vi "ZLIB Enumerate File Contents Old__ogtk.vi"(8 "error in (no error)":errorcluster, 11 "unzip Refnum":T2) -> (0 "error out":errorcluster, 1 "file infos":T1[](array[typedef]) {"file timestamp" format="%<%H:%M:%S\n%d/%m/%Y>T"; "external fa" format="%.0x"; "internal fa" format="%.0x"; "crc" format="%.0x"}, 2 "file names":string[](array[string]), 3 "unzip Refnum out":T2, 4 "file comments":string[](array[string]), 5 "extra data":string[](array[string]), 6 "global comment":string)   [LabVIEW 2020]
doc: "Lists all the information contained in the file of an unzip session."
uses:
  <userlib>/_OpenG.lib/lvzip/lvzip.llb/ZLIB Unzip Handle__ogtk.ctl
  <userlib>/_OpenG.lib/lvzip/lvzip.llb/ZLIB File Info Old__ogtk.ctl
panel:
  in  "file info":T1 {"file timestamp" format="%<%H:%M:%S\n%d/%m/%Y>T"; "external fa" format="%.0x"; "internal fa" format="%.0x"; "crc" format="%.0x"}
  # "Please visit http://www.OpenG.org to learn about the\nOpen Source LabVIEW software movement.\n\nNOTICE -- YOU MUST LEAVE THIS NOTICE IN PLACE.  PER THE TERMS OF THE LICENSE BELOW, YOU MAY SUBLICENSE THIS SOFTWARE \nIN ANY WAY THAT DOES NOT CONFLICT WITH THIS LICENSE.\n\n### BSD License (http://www.opensource.org/licenses/bsd-license.php) Begin ###\n \nCopyright (C) 2002-2004 Rolf Kalbermatter rolf.kalbermatter@citeng.com\nCopyright (C) 2002 Jim Kring jim@jimkring.com\n\nAll rights reserved.\n\nRedistribution and use in source and binary forms, with or without modification, are permitted provided that the following conditions are met:\n\n    * Redistributions of source code must retain the above copyright notice, this list of conditions and the following disclaimer.\n    * Redistributions in binary form must reproduce the above copyright notice, this list of conditions and the following disclaimer in the \n       documentation and/or other materials provided with the distribution.\n    * Neither the name of SciWare, James Kring, Inc., nor the names of its contributors may be used to endorse or promote products derived \n       from this software without specific prior written permission.\n\nTHIS SOFTWARE IS PROVIDED BY THE COPYRIGHT HOLDERS AND CONTRIBUTORS \"AS IS\" AND ANY EXPRESS OR IMPLIED WARRANTIES, \nINCLUDING, BUT NOT LIMITED TO, THE IMPLIED WARRANTIES OF MERCHANTABILITY AND FITNESS FOR A PARTICULAR PURPOSE ARE \nDISCLAIMED. IN NO EVENT SHALL THE COPYRIGHT OWNER OR CONTRIBUTORS BE LIABLE FOR ANY DIRECT, INDIRECT, INCIDENTAL,\n SPECIAL, EXEMPLARY, OR CONSEQUENTIAL DAMAGES (INCLUDING, BUT NOT LIMITED TO, PROCUREMENT OF SUBSTITUTE GOODS OR \nSERVICES; LOSS OF USE, DATA, OR PROFITS; OR BUSINESS INTERRUPTION) HOWEVER CAUSED AND ON ANY THEORY OF LIABILITY, \nWHETHER IN CONTRACT, STRICT LIABILITY, OR TORT (INCLUDING NEGLIGENCE OR OTHERWISE) ARISING IN ANY WAY OUT OF THE USE \nOF THIS SOFTWARE, EVEN IF ADVISED OF THE POSSIBILITY OF SUCH DAMAGE.\n\n### BSD License End ###"
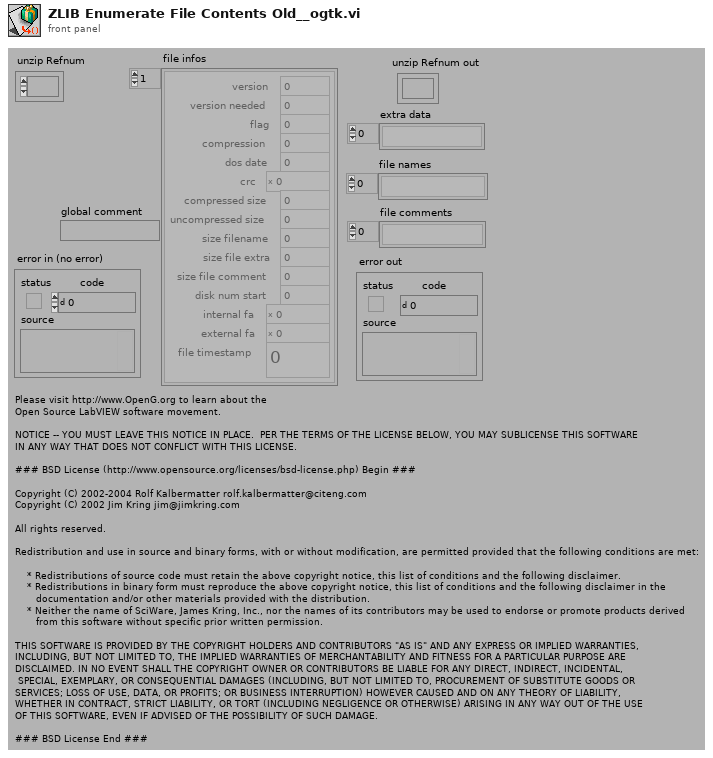
[diagram p1: front panel]
types:
  T1 = typedef "ZLIB File Info Old__ogtk.ctl" = cluster{"version":u32, "version needed":u32, "flag":u32, "compression":u32, "dos date":u32, "crc":u32, "compressed size":u32, "uncompressed size":u32, "size filename":u32, "size file extra":u32, "size file comment":u32, "disk num start":u32, "internal fa":u32, "external fa":u32, "file timestamp":u32}
  T2 = typedef "ZLIB Unzip Handle__ogtk.ctl" = refnum<k1>
  T3 = typedef "ZLIB File Info__ogtk.ctl" = cluster{"version":u32, "version needed":u32, "encrypted":bool, "flag":u32, "compression":i32, "dos date":u32, "crc":u32, "compressed size":u32, "uncompressed size":u32, "extra info":string, "file comment":string, "disk num start":u32, "internal fa":u32, "external fa":u32, "file timestamp":u32}
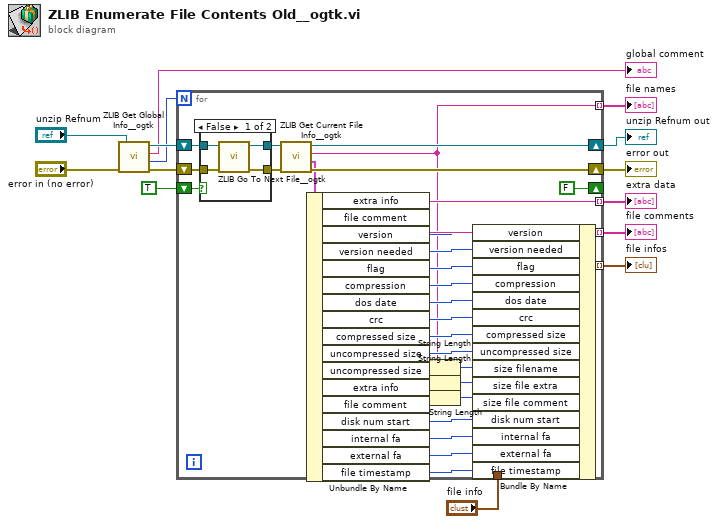
[diagram p0: block diagram]
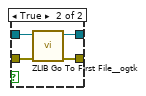
[diagram p2: hidden frame]
diagram:
  n1 = call <userlib>:"ZLIB Get Global Info__ogtk.vi"("error in (no error)"="error in (no error)", "unzip Refnum"="unzip Refnum") -> ("error out"=w14:errorcluster, "nEntry"=w1:u32, "global comment"=→"global comment":string, "unzip Refnum out"=w13:T2)  [unwired: 2 in]
  n2 = for {
    N: w1 -> [_]
    shift-right: [w38] -> w6
    shift-left: w13 -> [w44]
    shift-right: [w39] -> w5
    shift-left: w14 -> [w43]
    shift-right: [FALSE] -> _
    shift-left: TRUE -> [w45]
    tunnel: [w19] -> w11 mode=indexing
    tunnel: [w36] -> w10 mode=indexing
    tunnel: [w33] -> w9 mode=indexing
    tunnel: [w35] -> w4 mode=indexing
    tunnel: "file info" -> [w34]
    n3 = case shown="False" w45 {
      tunnel: w44 -> [w48 w53]
      tunnel: w43 -> [w49 w52]
      tunnel: [w47 w51] -> w41
      tunnel: [w46 w50] -> w42
      frame False {
        n4 = call <userlib>:"ZLIB Go To Next File__ogtk.vi"("error in (no error)"=w49, "unzip Refnum"=w48) -> ("error out"=w46:errorcluster, "unzip Refnum out"=w47:T2)  [unwired: 4 in]
      }
      frame True {
        n5 = call <userlib>:"ZLIB Go To First File__ogtk.vi"("error in (no error)"=w52, "unzip Refnum"=w53) -> ("error out"=w50:errorcluster, "unzip Refnum out"=w51:T2)  [unwired: 4 in]
      }
    }
    n6 = call <userlib>:"ZLIB Get Current File Info__ogtk.vi"("error in (no error)"=w42, "unzip Refnum"=w41) -> ("error out"=w39:errorcluster, "file info"=w37:T3, "name"=w19:string, "unzip Refnum out"=w38:T2)  [unwired: 6 in]
    n7 = Unbundle By Name(w37) -> ("extra info"=w35:string, "file comment"=w36:string, "version"=w32:u32, "version needed"=w31:u32, "flag"=w30:u32, "compression"=w29:i32, "dos date"=w28:u32, "crc"=w27:u32, "compressed size"=w26:u32, "uncompressed size"=w25:u32, "extra info"=w17:string, "file comment"=w18:string, "disk num start"=w24:u32, "internal fa"=w23:u32, "external fa"=w22:u32, "file timestamp"=w21:u32)  [unwired: 1 out]
    n8 = String Length(string=w19) -> (length=w20:i32)
    n9 = String Length(string=w17) -> (length=w15:i32)
    n10 = String Length(string=w18) -> (length=w16:i32)
    n11 = Bundle By Name(cluster=w34, "version"=w32, "version needed"=w31, "flag"=w30, "compression"=w29, "dos date"=w28, "crc"=w27, "compressed size"=w26, "uncompressed size"=w25, "size filename"=w20, "size file extra"=w15, "size file comment"=w16, "disk num start"=w24, "internal fa"=w23, "external fa"=w22, "file timestamp"=w21) -> (w33:T1)
  }
  "file names" <- w11
  "file comments" <- w10
  "file infos" <- w9
  "error out" <- w5
  "unzip Refnum out" <- w6
  "extra data" <- w4
